vi "Make Commands Absolute.vi"(8 "error in (no error)":errorcluster, 11 "Tool Path in":refnum<class "Tool Path.lvclass">) -> (0 "error out":errorcluster, 3 "Tool Path out":refnum<class "Tool Path.lvclass">)   [LabVIEW 2019, in "Tool Path.lvclass"]
uses:
  Tool Path.lvclass
  Parse/ParsePaths/Path.lvclass
  Parse/PathCommands/PathCommands.lvclass
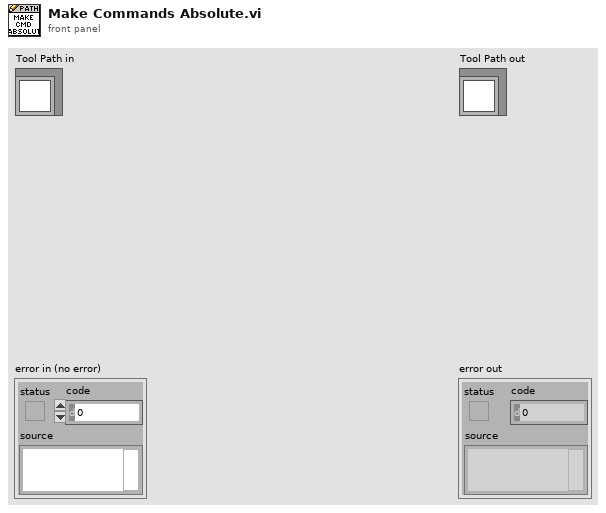
[diagram p1: front panel]
types:
  T1 = typedef "PathCommands.lvclass/Point.ctl" = cluster{"X":dbl, "Y":dbl}
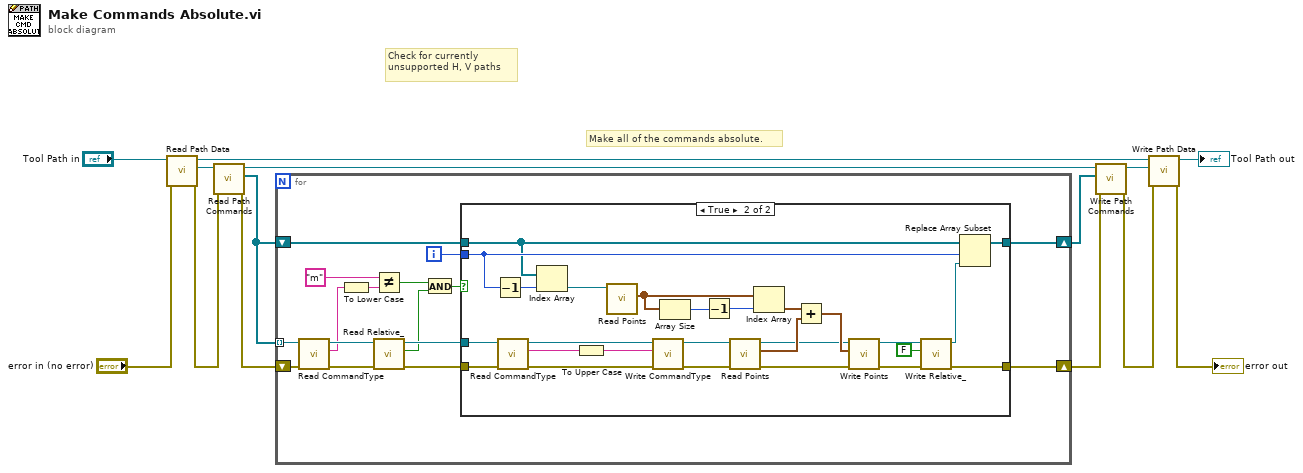
[diagram p0: block diagram]
diagram:
  # "Check for currently unsupported H, V paths"
  # "Make all of the commands absolute."
  n1 = call-dynamic "Read Path Data.vi"("error in (no error)"="error in (no error)", "Tool Path in"="Tool Path in") -> ("error out"=w3:errorcluster, "Path.lvclass"=w8:refnum<class "Path.lvclass">, "Tool Path out"=w7:refnum<class "Tool Path.lvclass">)  [unwired: 7 in]
  n2 = call "Read Path Commands.vi"("error in (no error)"=w3, "Path in"=w8) -> ("error out"=w13:errorcluster, "Path Commands"=w14:refnum<class "PathCommands.lvclass">[], "Path out"=w12:refnum<class "Path.lvclass">)  [unwired: 7 in]
  n3 = for {
    tunnel: w14 -> [w26] mode=indexing
    shift-right: [w17] -> w11
    shift-left: w13 -> [w16]
    shift-right: [w15] -> w10
    shift-left: w14 -> [w29]
    i -> [w28]
    n4 = call-dynamic "Read CommandType.vi"("error in (no error)"=w16, "PathCommands in"=w26) -> ("error out"=w19:errorcluster, "CommandType"=w20:string, "PathCommands out"=w27:refnum<class "PathCommands.lvclass">)  [unwired: 7 in]
    n5 = To Lower Case(string=w20) -> (all lower case string=w24:string)
    n6 = Not Equal?(x="m", y=w24) -> (x != y?=w22:bool)
    n7 = call-dynamic "Read Relative_.vi"("error in (no error)"=w19, "PathCommands in"=w27) -> ("error out"=w18:errorcluster, "Relative?"=w21:bool, "PathCommands out"=w30:refnum<class "PathCommands.lvclass">)  [unwired: 7 in]
    n8 = And(x=w22, y=w21) -> (x .and. y?=w25:bool)
    n9 = case shown="True" w25 {
      tunnel: w30 -> [_ w44]
      tunnel: w29 -> [w31 w33]
      tunnel: w28 -> [_ w34]
      tunnel: w18 -> [w32 w39]
      tunnel: [w32 w37] -> w17
      tunnel: [w31 w35] -> w15
      frame False {
      }
      frame True {
        n10 = Decrement(x=w34) -> (x-1=w58:i32)
        n11 = call-dynamic "Read CommandType.vi"("error in (no error)"=w39, "PathCommands in"=w44) -> ("error out"=w41:errorcluster, "CommandType"=w43:string, "PathCommands out"=w46:refnum<class "PathCommands.lvclass">)  [unwired: 7 in]
        n12 = Index Array(array=w33, index=w58) -> (element=w57:refnum<class "PathCommands.lvclass">)
        n13 = To Upper Case(1:w43) -> (0:w42:string)
        n14 = call-dynamic "Read Points.vi"("PathCommands in"=w57) -> ("Points"=w55:T1[])  [unwired: 8 in, 2 out]
        n15 = call-dynamic "Write CommandType.vi"("error in (no error)"=w41, "CommandType"=w42, "PathCommands in"=w46) -> ("error out"=w40:errorcluster, "PathCommands out"=w45:refnum<class "PathCommands.lvclass">)  [unwired: 7 in]
        n16 = Array Size(array=w55) -> (size(s)=w56:i32)
        n17 = Decrement(x=w56) -> (x-1=w54:i32)
        n18 = call-dynamic "Read Points.vi"("error in (no error)"=w40, "PathCommands in"=w45) -> ("error out"=w38:errorcluster, "Points"=w52:T1[], "PathCommands out"=w47:refnum<class "PathCommands.lvclass">)  [unwired: 7 in]
        n19 = Index Array(array=w55, index=w54) -> (element=w53:T1)
        n20 = Add(x=w53, y=w52) -> (x+y=w51:T1[])
        n21 = call-dynamic "Write Points.vi"("error in (no error)"=w38, "Points"=w51, "PathCommands in"=w47) -> ("error out"=w48:errorcluster, "PathCommands out"=w50:refnum<class "PathCommands.lvclass">)  [unwired: 7 in]
        n22 = call-dynamic "Write Relative_.vi"("error in (no error)"=w48, "Relative?"=FALSE, "PathCommands in"=w50) -> ("error out"=w37:errorcluster, "PathCommands out"=w36:refnum<class "PathCommands.lvclass">)  [unwired: 7 in]
        n23 = Replace Array Subset(array=w33, new element=w36, index=w34) -> (w35:refnum<class "PathCommands.lvclass">[])
      }
    }
  }
  n24 = call "Write Path Commands.vi"("error in (no error)"=w11, "Path Commands"=w10, "Path in"=w12) -> ("error out"=w2:errorcluster, "Path out"=w9:refnum<class "Path.lvclass">)  [unwired: 7 in]
  n25 = call-dynamic "Write Path Data.vi"("error in (no error)"=w2, "Path.lvclass"=w9, "Tool Path in"=w7) -> ("error out"=→"error out":errorcluster, "Tool Path out"=→"Tool Path out":refnum<class "Tool Path.lvclass">)  [unwired: 7 in]
